vi "Get Channel Name Core.vi"(8 "error in (no error)":errorcluster, 10 "channel index (1)":i32=1 caption="Channel Index (1)", 11 "IVI_DCPwr in":refnum<class "IVI_DCPwr.lvclass">) -> (0 "error out":errorcluster, 2 "channel name":string caption="Channel Name", 3 "IVI_DCPwr out":refnum<class "IVI_DCPwr.lvclass">)   [LabVIEW 2013, in "IVI_DCPwr.lvlib" / "IVI_DCPwr.lvclass"]
doc: "This VI returns the highest-level channel name that corresponds to the specific driver channel string that is in the channel table at an index you specify."
uses:
  IVI_DCPwr.lvclass
  IVI_DCPwr.lvclass/IVI_DCPwr.ctl
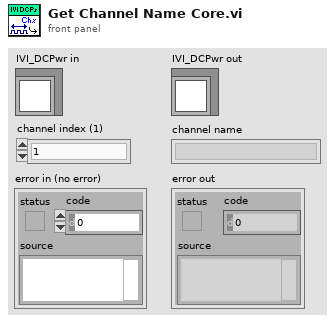
[diagram p1: front panel]
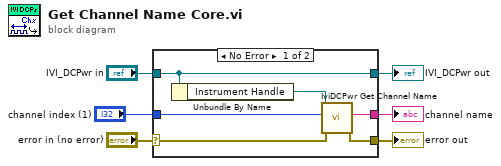
[diagram p0: block diagram]
diagram:
  n1 = case shown="No Error" "error in (no error)" {
    selector: "error in (no error)" -> [w10 w14]
    tunnel: [w9 w14] -> w5
    tunnel: [w12 w13] -> w3
    tunnel: "IVI_DCPwr in" -> [w12 w13]
    tunnel: "channel index (1)" -> [w8 _]
    tunnel: [w7 _] -> w1
    frame No Error {
      n2 = Unbundle By Name(w12) -> ("Instrument Handle"=w11:refnum<k15>)
      n3 = call <vilib>:"IviDCPwr Get Channel Name.vi"("error in (no error)"=w10, "channel index (1)"=w8, "instrument handle"=w11) -> ("error out"=w9:errorcluster, "channel name"=w7:string)  [unwired: 6 in, 1 out]
    }
    frame Error {
    }
  }
  "error out" <- w5
  "IVI_DCPwr out" <- w3
  "channel name" <- w1
